vi "Determine Warnings Modified.vi"() -> ()   [LabVIEW 2014]
panel:
  in  "Currnet Temp 2":dbl
  out "Warning Text":string
  out "Warning?":bool
  in  "Min Temp":dbl
  in  "Max Temp":dbl
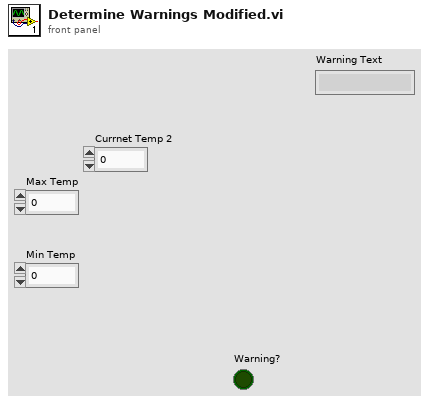
[diagram p1: front panel]
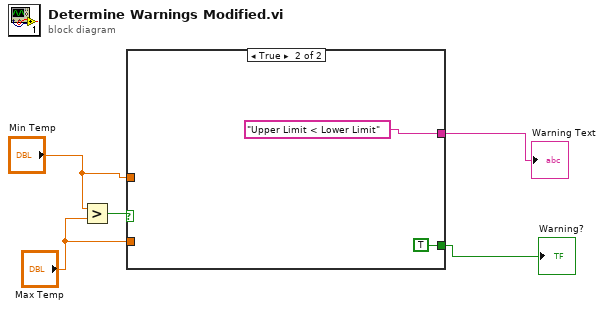
[diagram p0: block diagram]
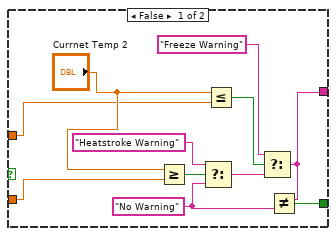
[diagram p2: hidden frame]
diagram:
  n1 = Greater?(x="Min Temp", y="Max Temp") -> (0:w5:bool)
  n2 = case shown="True" w5 {
    tunnel: "Max Temp" -> [w10 _]
    tunnel: "Min Temp" -> [w8 _]
    tunnel: [w7 "Upper Limit < Lower Limit"] -> w2
    tunnel: [w6 TRUE] -> w1
    frame False {
      w16 = "No Warning"
      n3 = Greater Or Equal?(x="Currnet Temp 2", y=w10) -> (x >= y?=w12:bool)
      n4 = Select(t="Heatstroke Warning", s=w12, f=w16) -> (s? t:f=w14:string)
      n5 = Less Or Equal?(x="Currnet Temp 2", y=w8) -> (x <= y?=w11:bool)
      n6 = Select(t="Freeze Warning", s=w11, f=w14) -> (s? t:f=w7:string)
      n7 = Not Equal?(x=w7, y=w16) -> (x != y?=w6:bool)
    }
    frame True {
    }
  }
  "Warning?" <- w1
  "Warning Text" <- w2
